vi "example.vi"() -> ()   [LabVIEW 2016]
uses:
  Monochromator/Monochromator.lvclass
  MonoPubSubData/MonoPubSubData.lvclass
  Typedefs/SlitType.ctl
  Typedefs/slit.ctl
  Typedefs/slitWidth.ctl
  Typedefs/wavelength.ctl
  Typedefs/GratingType.ctl
panel:
  out "GratingType":T1
  out "slitPosition":T2
  out "wavelength":T5
  in  "stop":bool
  in  "getWavelength":bool
  in  "getSlitPosition":bool
  in  "GetGrating":bool
  in  "sendGratingType":bool
  in  "sendSlitPosition":bool
  in  "sendWavelength":bool
  in  "GratingType":T1
  in  "slitPosition":T2
  in  "wavelength":T5
  # "Wavelength"
  # "Device Status"
  # "Slit"
  # "Slit"
  # "Grating"
  # "Grating"
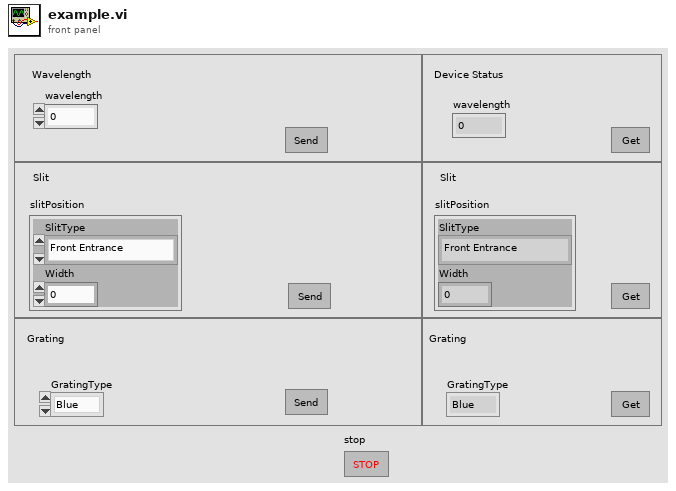
[diagram p1: front panel]
types:
  T1 = typedef "GratingType.ctl" = enum16{"Blue", "Red", "Mirror"}
  T2 = typedef "slit.ctl" = cluster{"SlitType":T3, "Width":T4}
  T3 = typedef "SlitType.ctl" = enum16{"Front Entrance", "Side Entrance", "Front Exit", "Side Exit", "First Intermediate", "Second Intermediate"}
  T4 = typedef "slitWidth.ctl" = dbl
  T5 = typedef "wavelength.ctl" = dbl
  T6 = typedef "slitPosition.ctl" = dbl
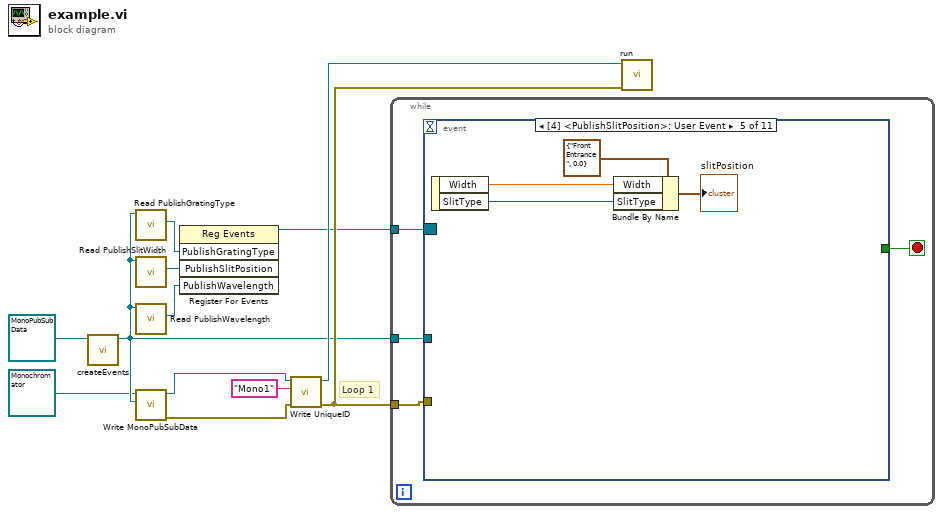
[diagram p0: block diagram]
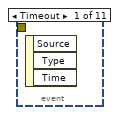
[diagram p2: hidden frame]
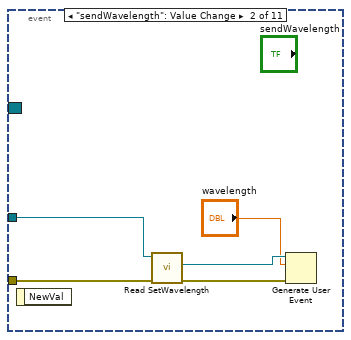
[diagram p3: hidden frame]
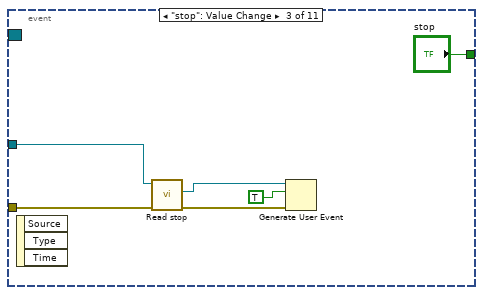
[diagram p4: hidden frame]
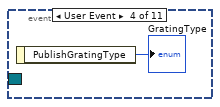
[diagram p5: hidden frame]
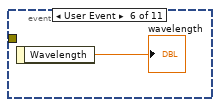
[diagram p6: hidden frame]
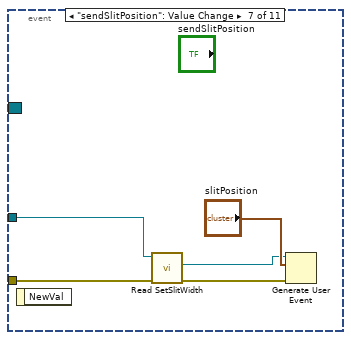
[diagram p7: hidden frame]
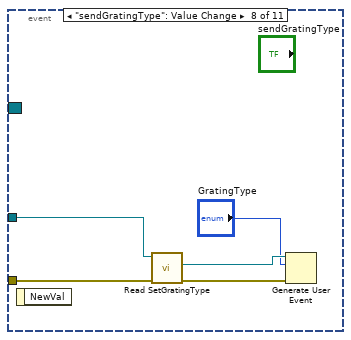
[diagram p8: hidden frame]
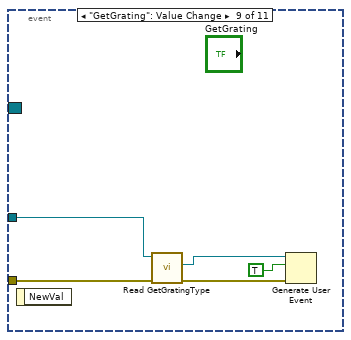
[diagram p9: hidden frame]
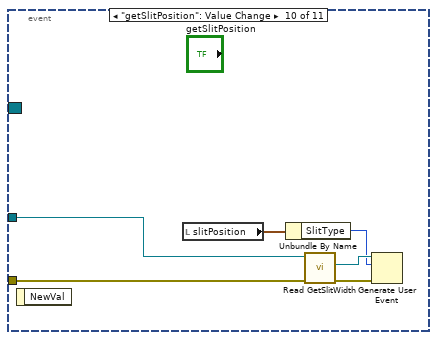
[diagram p10: hidden frame]
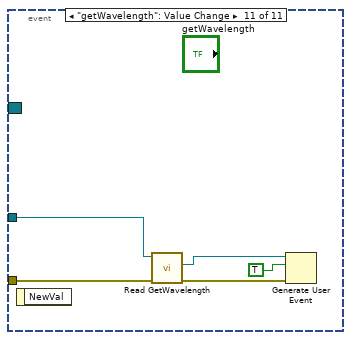
[diagram p11: hidden frame]
diagram:
  # "Loop 1"
  n1 = call "createEvents.vi"("MonoPubSubData in"=refnum<class "MonoPubSubData.lvclass"> refnum ("MonoPubSubData.lvclass")) -> ("MonoPubSubData out"=w3:refnum<class "MonoPubSubData.lvclass">)  [unwired: 9 in, 1 out]
  n2 = call "Read PublishGratingType.vi"("MonoPubSubData in"=w3) -> ("PublishGratingType"=w4:refnum<user-event>)  [unwired: 8 in, 2 out]
  n3 = call "Read PublishSlitWidth.vi"("MonoPubSubData in"=w3) -> ("PublishSlitPosition"=w5:refnum<user-event>)  [unwired: 8 in, 2 out]
  n4 = call "Read PublishWavelength.vi"("MonoPubSubData in"=w3) -> ("PublishWavelength"=w6:refnum<user-event>)  [unwired: 8 in, 2 out]
  n5 = call "Write MonoPubSubData.vi"("MonoPubSubData.lvclass"=w3, "Monochromator in"=refnum<class "Monochromator.lvclass"> refnum ("Monochromator.lvclass")) -> ("error out"=w9:errorcluster, "Monochromator out"=w11:refnum<class "Monochromator.lvclass">)  [unwired: 8 in]
  n6 = register-events(w4, w5, w6) -> (reference out=w2:refnum<event-registration>)  [unwired: 2 in, 1 out]
  n7 = call "Write UniqueID.vi"("error in (no error)"=w9, "UniqueID"="Mono1", "Monochromator in"=w11) -> ("error out"=w8:errorcluster, "Monochromator out"=w7:refnum<class "Monochromator.lvclass">)  [unwired: 7 in]
  n8 = while {
    tunnel: w8 -> [w14]
    tunnel: w3 -> [w16]
    tunnel: w2 -> [w13]
    stop <- w15 stop-if-true
    n9 = event shown="[4] <PublishSlitPosition>: User Event" {
      selector: w13 -> [_ _ _ _ _ _ _ _ _ _ _]
      dyn-events: _ -> [_ _ _ _ _ _ _ _ _ _ _]
      timeout: _ -> [_ _ _ _ _ _ _ _ _ _ _]
      tunnel: w16 -> [_ w21 w26 _ _ _ w37 w42 w47 w53 w59]
      tunnel: [_ _ "stop" _ _ _ _ _ _ _ _] -> w15
      tunnel: w14 -> [_ w20 w23 _ _ _ w38 w43 w48 w54 w56]
      event Timeout {
        n10 = event-data() -> ()  [unwired: 1 in, 3 out]
      }
      event "sendWavelength": Value Change {
        n11 = event-data() -> ()  [unwired: 1 in, 1 out]
        n12 = call "Read SetWavelength.vi"("error in (no error)"=w20, "MonoPubSubData in"=w21) -> ("error out"=w17:errorcluster, "SetWavelength"=w19:refnum<user-event>)  [unwired: 7 in, 1 out]
        n13 = Generate User Event(user event=w19, event data cluster="wavelength", error in=w17) -> ()  [unwired: 1 in, 2 out]
      }
      event "stop": Value Change {
        n14 = event-data() -> ()  [unwired: 1 in, 3 out]
        n15 = call "Read stop.vi"("error in (no error)"=w23, "MonoPubSubData in"=w26) -> ("error out"=w22:errorcluster, "stop"=w25:refnum<user-event>)  [unwired: 7 in, 1 out]
        n16 = Generate User Event(user event=w25, event data cluster=TRUE ("event data"), error in=w22) -> ()  [unwired: 1 in, 2 out]
      }
      event User Event {
        n17 = event-data() -> ("PublishGratingType"=→"GratingType":T1)  [unwired: 1 in]
      }
      event User Event {
        n18 = event-data() -> ("Width"=w30:T6, "SlitType"=w31:T3)  [unwired: 1 in]
        n19 = Bundle By Name(cluster=T2 {"SlitType"=enum."Front Entrance", "Width"=0.0} ("slitPosition 2"), "Width"=w30, "SlitType"=w31) -> (→"slitPosition":T2)
      }
      event User Event {
        n20 = event-data() -> ("Wavelength"=→"wavelength":T5)  [unwired: 1 in]
      }
      event "sendSlitPosition": Value Change {
        n21 = event-data() -> ()  [unwired: 1 in, 1 out]
        n22 = call "Read SetSlitWidth.vi"("error in (no error)"=w38, "MonoPubSubData in"=w37) -> ("error out"=w34:errorcluster, "SetSlitPosition"=w35:refnum<user-event>)  [unwired: 7 in, 1 out]
        n23 = Generate User Event(user event=w35, event data cluster="slitPosition", error in=w34) -> ()  [unwired: 1 in, 2 out]
      }
      event "sendGratingType": Value Change {
        n24 = event-data() -> ()  [unwired: 1 in, 1 out]
        n25 = call "Read SetGratingType.vi"("error in (no error)"=w43, "MonoPubSubData in"=w42) -> ("error out"=w39:errorcluster, "SetGratingType"=w41:refnum<user-event>)  [unwired: 7 in, 1 out]
        n26 = Generate User Event(user event=w41, event data cluster="GratingType", error in=w39) -> ()  [unwired: 1 in, 2 out]
      }
      event "GetGrating": Value Change {
        n27 = event-data() -> ()  [unwired: 1 in, 1 out]
        n28 = call "Read GetGratingType.vi"("error in (no error)"=w48, "MonoPubSubData in"=w47) -> ("error out"=w44:errorcluster, "GetGratingType"=w46:refnum<user-event>)  [unwired: 7 in, 1 out]
        n29 = Generate User Event(user event=w46, event data cluster=TRUE ("event data"), error in=w44) -> ()  [unwired: 1 in, 2 out]
      }
      event "getSlitPosition": Value Change {
        n30 = event-data() -> ()  [unwired: 1 in, 1 out]
        n31 = local read "slitPosition"() -> (w50:T2)
        n32 = Unbundle By Name(w50) -> ("SlitType"=w49:T3)
        n33 = call "Read GetSlitWidth.vi"("error in (no error)"=w54, "MonoPubSubData in"=w53) -> ("error out"=w51:errorcluster, "GetSlitPosition"=w52:refnum<user-event>)  [unwired: 7 in, 1 out]
        n34 = Generate User Event(user event=w52, event data cluster=w49, error in=w51) -> ()  [unwired: 1 in, 2 out]
      }
      event "getWavelength": Value Change {
        n35 = event-data() -> ()  [unwired: 1 in, 1 out]
        n36 = call "Read GetWavelength.vi"("error in (no error)"=w56, "MonoPubSubData in"=w59) -> ("error out"=w55:errorcluster, "GetWavelength"=w58:refnum<user-event>)  [unwired: 7 in, 1 out]
        n37 = Generate User Event(user event=w58, event data cluster=TRUE ("event data"), error in=w55) -> ()  [unwired: 1 in, 2 out]
      }
    }
  }
  n38 = call "run.vi"("error in (no error)"=w8, "Monochromator in"=w7) -> ()  [unwired: 8 in, 2 out]
